vi "ROI grp-Delete selected ROIs from group.vi"(8 "error in (no error)":errorcluster, 10 "ROI number of ROIs deleted from each group.":T1(array[cluster])) -> (0 "error out":errorcluster)   [LabVIEW 2013]
uses:
  Typedefs/Get-Set-Clear Control.ctl
  Program Files (x86)/National Instruments/LabVIEW 2013/user.lib/_OpenG.lib/array/array.llb/Delete Elements from 1D Array (I32)__ogtk.vi
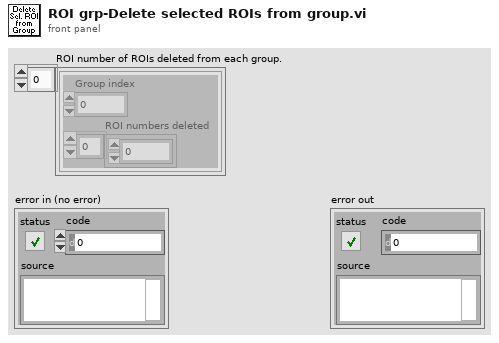
[diagram p1: front panel]
types:
  T1 = cluster{"Group index":i32, "ROI numbers deleted":i32[]}[]
  T2 = typedef "Get-Set-Clear Control.ctl" = enum16{"Get", "Set", "Clear"}
  T3 = typedef "ROI group info cluster.ctl" = cluster{"Group name":string, "# ROI in group":i32, "ROI numbers in group":i32[], "Group region specifier cluster":T4}
  T4 = typedef "ROI Descriptor" = cluster{"Global Rectangle":i32[], "Contours":cluster{"ID":enum32{"External", "Internal"}, "Type":u32, "Coordinates":i32[]}[]}
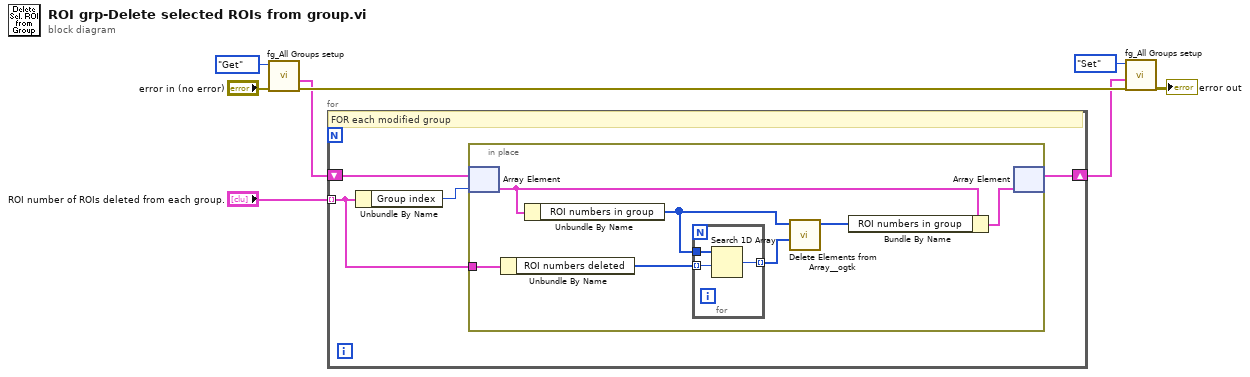
[diagram p0: block diagram]
diagram:
  n1 = call "fg_All Groups setup.vi"("error in (no error)"="error in (no error)", "Function"=Get-Set-Clear_Control."Get") -> ("error out"=w8:errorcluster, "Groups setup out"=w4:T3[])  [unwired: 8 in]
  n2 = for {
    tunnel: "ROI number of ROIs deleted from each group." -> [w9] mode=indexing
    shift-right: [w11] -> w6
    shift-left: w4 -> [w12]
    # "FOR each modified group"
    n3 = Unbundle By Name(w9) -> ("Group index"=w10:i32)
    n4 = in-place {
      in-place-border: w9 -> [w18]
      n5 = in-place-array #1(w12, w10) -> (w17:T3)
      n6 = Unbundle By Name(w18) -> ("ROI numbers deleted"=w13:i32[])
      n7 = Unbundle By Name(w17) -> ("ROI numbers in group"=w14:i32[])
      n8 = for {
        tunnel: [w22] -> w16 mode=indexing
        tunnel: w14 -> [w21]
        tunnel: w13 -> [w20] mode=indexing
        n9 = Search 1D Array(1D array=w21, element=w20) -> (index of element=w22:i32)  [unwired: 1 in]
      }
      n10 = call-poly "Delete Elements from Array__ogtk.vi"("indices"=w16, "array"=w14) -> ("array w/ subset deleted"=w15:i32[])  [unwired: 8 in, 1 out]
      n11 = Bundle By Name(cluster=w17, "ROI numbers in group"=w15) -> (w19:T3)
      n12 = in-place-array #1(w19) -> (w11:T3[])  [unwired: 1 out]
    }
  }
  n13 = call "fg_All Groups setup.vi"("error in (no error)"=w8, "Groups setup in"=w6, "Function"=Get-Set-Clear_Control."Set") -> ("error out"=→"error out":errorcluster)  [unwired: 7 in, 1 out]
